vi "detector-init.vi"(5 "Cooling Set":T1={"iDus"=TRUE, "idus-temp"=-90, "Newton"=TRUE, "newton-temp"=-70, "Clara"=TRUE, "clara-temp"=-55, "Xeva"=TRUE, "xeva-temp"=-55} {"xeva-temp" min=-55 max=20 step=5; "clara-temp" min=-55 max=20 step=5; "newton-temp" min=-90 max=20 step=5; "idus-temp" min=-90 max=20 step=5}) -> (0 "Status":T3={"Newton Init"=FALSE, "Newton Cooling"=FALSE, "Newton Parameters "=FALSE, "iDus Init"=FALSE, "iDus Cooling"=FALSE, "iDus Parameters"=FALSE, "Clara Init"=FALSE, "Clara Cooling"=FALSE, "Clara Parameters"=FALSE, "Newton Cooler StatusCode"=enum."DRV_TEMPERATURE_NOT_SUPPORTED", "iDus Cooler StatusCode"=enum."DRV_TEMPERATURE_NOT_SUPPORTED", "Clara Cooler StatusCode"=enum."DRV_TEMPERATURE_NOT_SUPPORTED"} caption="Status Cluster", 1 "cameras initialized":bool, 2 "Handle Cluster":cluster{"iDus":i32, "Newton":i32, "Clara":i32}, 3 "Detector Output Values":cluster{"iDus":i32, "Newton":i32, "Clara":i32}={"iDus"=25, "Newton"=25, "Clara"=25} caption="Detector Temperature Cluster")   [LabVIEW 2015]
uses:
  <userlib>/atmcd32d.llb/Error Code Enum typedef.ctl
  <userlib>/atmcd32d.llb/ReadMode_mode typedef.ctl
  <userlib>/atmcd32d.llb/AcquisitionMode_mode typedef.ctl
  <userlib>/atmcd32d.llb/TriggerMode_mode typedef.ctl
  <userlib>/atmcd32d.llb/HSSpeed_type typedef.ctl
  <userlib>/atmcd32d.llb/OutputAmplifier_type typedef.ctl
panel:
  out "Clara Error":errorcluster
  out "iDus Error":errorcluster
  out "Newton Error":errorcluster
  out "totalCameras":i32
  # "Init"
  # "Cooling"
  # "Parameters"
  # "Newton"
  # "iDus"
  # "Clara"
  # "Clara"
  # "iDus"
  # "Newton"
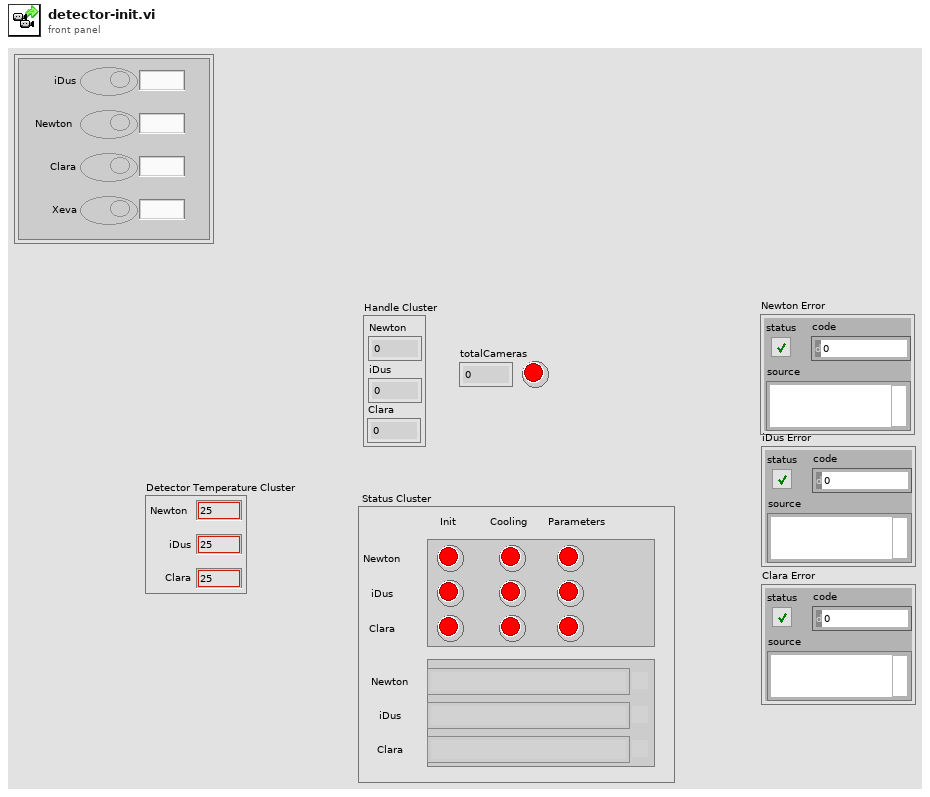
[diagram p1: front panel]
types:
  T1 = cluster{"iDus":bool, "idus-temp":i32, "Newton":bool, "newton-temp":i32, "Clara":bool, "clara-temp":i32, "Xeva":bool, "xeva-temp":i32}
  T2 = typedef "Error Code Enum typedef.ctl" = enum32{"N/A (0)", "DRV_ERROR_CODES", "DRV_SUCCESS", "DRV_VXDNOTINSTALLED", "DRV_ERROR_SCAN", "DRV_ERROR_CHECK_SUM", "DRV_ERROR_FILELOAD", "DRV_UNKNOWN_FUNC", "DRV_ERROR_VXD_INIT", "DRV_ERROR_ADDRESS", "DRV_ERROR_PAGELOCK", "DRV_ERROR_PAGEUNLOCK", "DRV_ERROR_BOARDTEST", "DRV_ERROR_ACK", "DRV_ERROR_UP_FIFO", "DRV_ERROR_PATTERN", "N/A (16)", "DRV_ACQUISITION_ERRORS", "DRV_ACQ_BUFFER", "DRV_ACQ_DOWNFIFO_FULL", "DRV_PROC_UNKONWN_INSTRUCTION", "DRV_ILLEGAL_OP_CODE", "DRV_KINETIC_TIME_NOT_MET", "DRV_ACCUM_TIME_NOT_MET", "DRV_NO_NEW_DATA", "N/A (25)", "DRV_SPOOLERROR", "N/A (27)", "N/A (28)", "N/A (29)", "N/A (30)", "N/A (31)", "N/A (32)", "DRV_TEMPERATURE_CODES", "DRV_TEMPERATURE_OFF", "DRV_TEMPERATURE_NOT_STABILIZED", "DRV_TEMPERATURE_STABILIZED", "DRV_TEMPERATURE_NOT_REACHED", "DRV_TEMPERATURE_OUT_RANGE", "DRV_TEMPERATURE_NOT_SUPPORTED", "DRV_TEMPERATURE_DRIFT", "N/A (41)", "N/A (42)", "N/A (43)", "N/A (44)", "N/A (45)", "N/A (46)", "N/A (47)", "N/A (48)", "DRV_GENERAL_ERRORS", "DRV_INVALID_AUX", "DRV_COF_NOTLOADED", "DRV_FPGAPROG", "DRV_FLEXERROR", "DRV_GPIBERROR", "N/A (55)", "N/A (56)", "N/A (57)", "N/A (58)", "N/A (59)", "N/A (60)", "N/A (61)", "N/A (62)", "N/A (63)", "DRV_DATATYPE", "DRV_DRIVER_ERRORS", "DRV_P1INVALID", "DRV_P2INVALID", "DRV_P3INVALID", "DRV_P4INVALID", "DRV_INIERROR", "DRV_COFERROR", "DRV_ACQUIRING", "DRV_IDLE", "DRV_TEMPCYCLE", "DRV_NOT_INITIALIZED", "DRV_P5INVALID", "DRV_P6INVALID", "DRV_INVALID_MODE", "DRV_INVALID_FILTER", "DRV_I2CERRORS", "DRV_I2CDEVNOTFOUND", "DRV_I2CTIMEOUT", "DRV_P7INVALID", "N/A (84)", "N/A (85)", "N/A (86)", "N/A (87)", "N/A (88)", "N/A (89)", "DRV_IOCERROR", "DRV_VRMVERSIONERROR"}
  T3 = cluster{"Newton Init":bool, "Newton Cooling":bool, "Newton Parameters ":bool, "iDus Init":bool, "iDus Cooling":bool, "iDus Parameters":bool, "Clara Init":bool, "Clara Cooling":bool, "Clara Parameters":bool, "Newton Cooler StatusCode":T2, "iDus Cooler StatusCode":T2, "Clara Cooler StatusCode":T2}
  T4 = cluster{"iDus Init":bool, "Newton Init":bool, "iDus Cooling":bool, "Newton Cooling":bool, "Clara Init":bool, "Clara Cooling":bool, "iDus Parameters":bool, "Newton Parameters ":bool, "Clara Parameters":bool, "Newton Cooler StatusCode":T2, "iDus Cooler StatusCode":T2, "Clara Cooler StatusCode":T2}
  T5 = cluster{"InGaAs Handle":i32, "CCD Handle":i32, "Clara Handle":i32}
  T6 = typedef "TriggerMode_mode typedef.ctl" = enum16{"Internal", "External", "N/A (2)", "N/A (3)", "N/A (4)", "N/A (5)", "External Start", "External Exposure (Bulb)", "N/A (8)", "External FVB EM", "Software", "N/A (11)", "External Charge Shifting"}
  T7 = typedef "AcquisitionMode_mode typedef.ctl" = enum16{"Reserved (0)", "Single Scan", "Accumulate", "Kinetics", "Fast Kinetics", "Run Till Abort", "Reserved (6)", "Reserved (7)", "Reserved (8)", "Time Delayed Integration"}
  T8 = typedef "ReadMode_mode typedef.ctl" = enum16{"Full Vertical Binning", "Multi-Track", "Random-Track", "Single-Track", "Image"}
  T9 = typedef "HSSpeed_type typedef.ctl" = enum16{"EM Amp", "Conventional Amp"}
  T10 = typedef "OutputAmplifier_type typedef.ctl" = enum16{"Standard EMCCD gain register", "Conventional CCD register"}
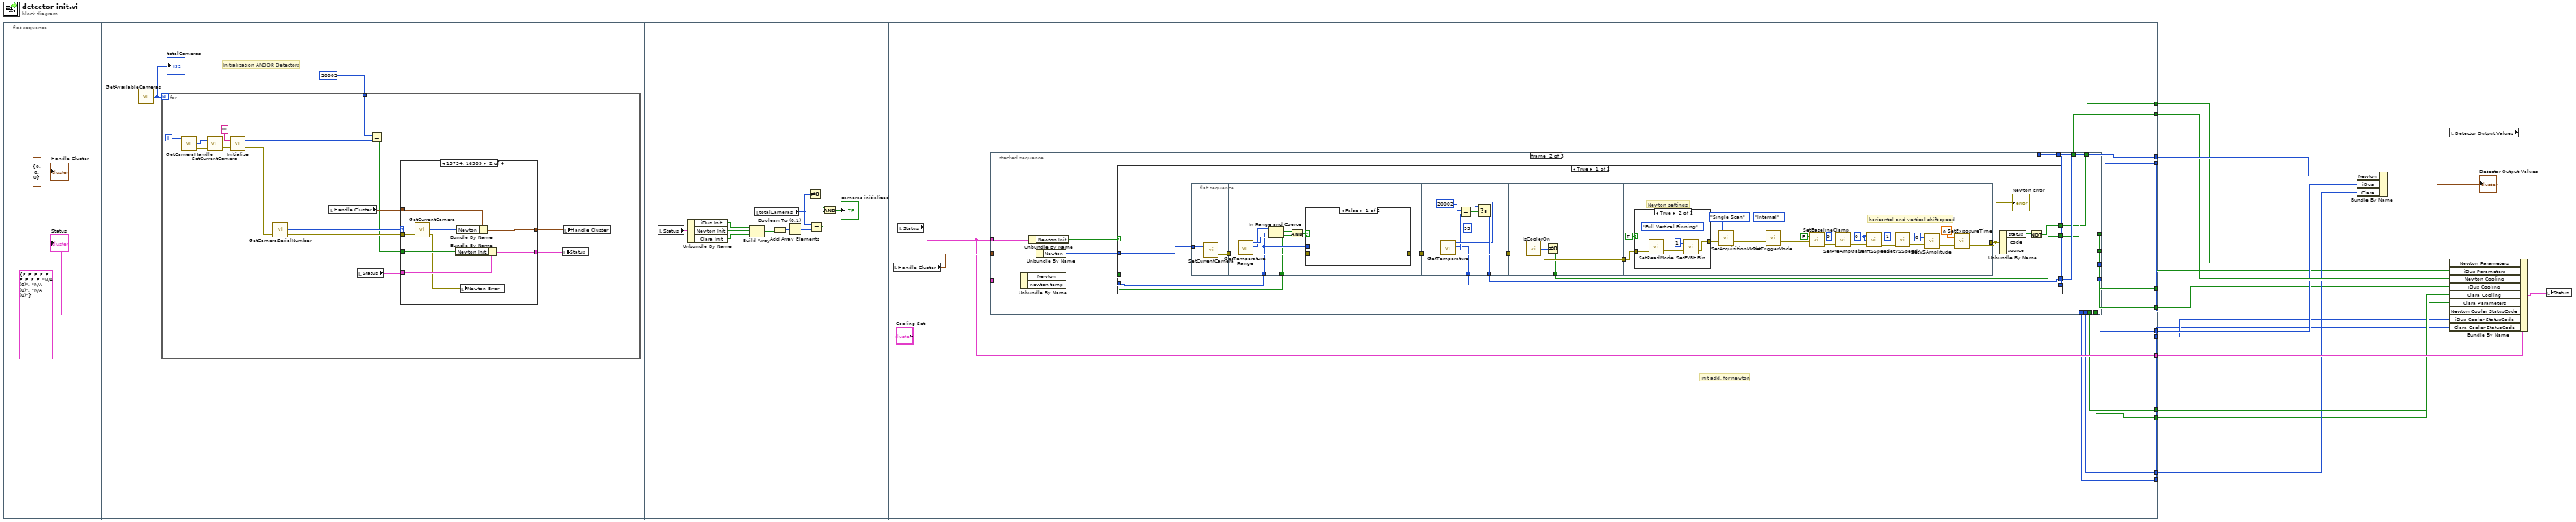
[diagram p0: block diagram]
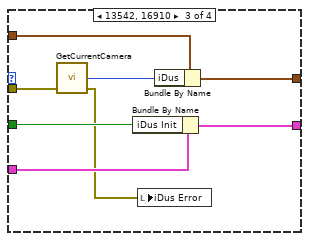
[diagram p3: hidden frame]
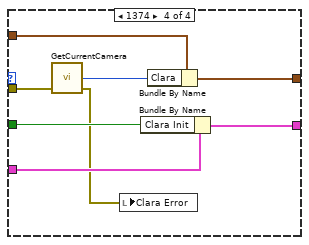
[diagram p4: hidden frame]
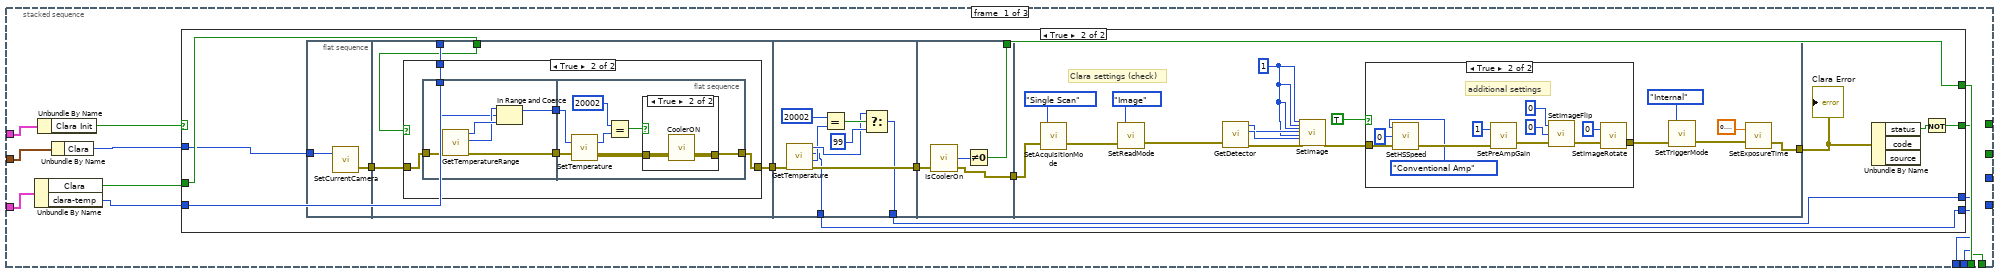
[diagram p5: hidden frame]
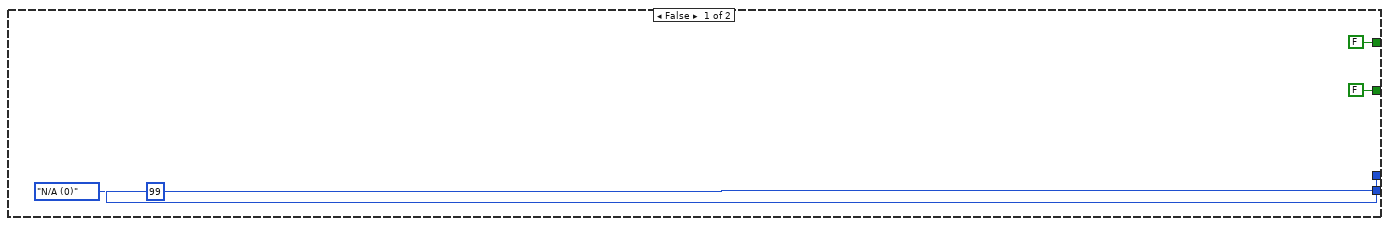
[diagram p6: hidden frame]
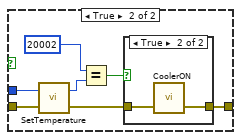
[diagram p10: hidden frame]
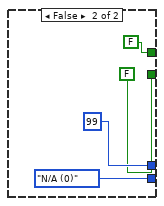
[diagram p13: hidden frame]
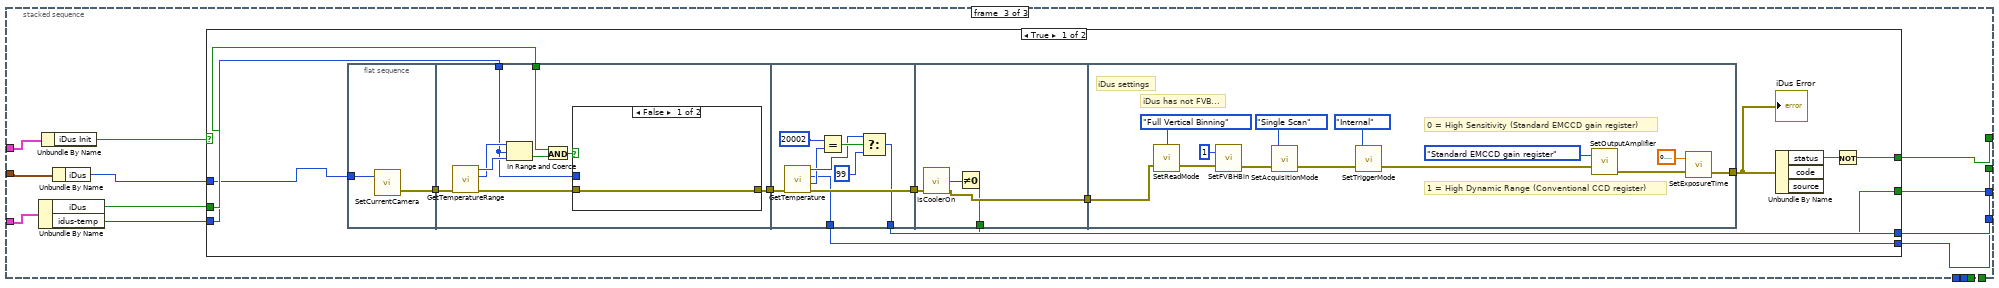
[diagram p14: hidden frame]
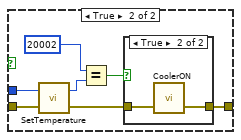
[diagram p15: hidden frame]
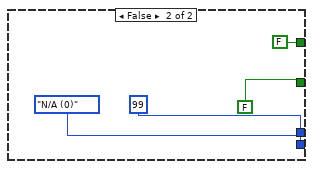
[diagram p17: hidden frame]
diagram:
  n1 = flat-sequence {
    tunnel: [w87] -> w13
    tunnel: [w85] -> w15
    tunnel: [w84] -> w12
    tunnel: [w77] -> w14
    tunnel: [w79] -> w9
    tunnel: [w75] -> w8
    tunnel: [w83] -> w7
    tunnel: [w78] -> w6
    tunnel: [w74] -> w5
    tunnel: [w82] -> w4
    tunnel: [w81] -> w3
    tunnel: [w80] -> w2
    tunnel: [w76] -> w1
    frame #0 {
      "Status" <- T4 {"iDus Init"=FALSE, "Newton Init"=FALSE, "iDus Cooling"=FALSE, "Newton Cooling"=FALSE, "Clara Init"=FALSE, "Clara Cooling"=FALSE, "iDus Parameters"=FALSE, "Newton Parameters "=FALSE, "Clara Parameters"=FALSE, "Newton Cooler StatusCode"=enum."N/A (0)", "iDus Cooler StatusCode"=enum."N/A (0)", "Clara Cooler StatusCode"=enum."N/A (0)"} ("Status")
      "Handle Cluster" <- T5 {"InGaAs Handle"=0, "CCD Handle"=0, "Clara Handle"=0} ("Handle Cluster")
    }
    frame #1 {
      # "Initialization ANDOR Detectors"
      n2 = call <userlib>:"GetAvailableCameras.vi"() -> ("totalCameras"=w20:i32)  [unwired: 3 in, 2 out]
      "totalCameras" <- w20
      n3 = for {
        N: w20 -> [_]
        tunnel: 20002 -> [w33]
        i -> [w28]
        n4 = call <userlib>:"GetCameraHandle.vi"("cameraIndex"=w28) -> ("error out"=w31:errorcluster, "cameraHandle"=w32:i32)  [unwired: 2 in, 1 out]
        n5 = call <userlib>:"SetCurrentCamera.vi"("error in (no error)"=w31, "cameraHandle"=w32) -> ("error out"=w30:errorcluster)  [unwired: 1 out]
        n6 = call <userlib>:"Initialize.vi"("error in (no error)"=w30, "directory (\"\")"="" ("directory (\"\")")) -> ("error out"=w29:errorcluster, "DLL error code"=w34:u32)
        n7 = call <userlib>:"GetCameraSerialNumber.vi"("error in (no error)"=w29) -> ("error out"=w25:errorcluster, "number"=w27:i32)  [unwired: 2 in, 1 out]
        n8 = local read "Handle Cluster"() -> (w26:cluster{"iDus":i32, "Newton":i32, "Clara":i32})
        n9 = local read "Status"() -> (w23:T3)
        n10 = Equal?(x=w33, y=w34) -> (x = y?=w21:bool)
        n11 = case shown="13734, 16909" w27 {
          tunnel: w26 -> [w37 w45 w50 w61]
          tunnel: w25 -> [_ w43 w53 w55]
          tunnel: [w37 w42 w51 w60] -> w24
          tunnel: w23 -> [w36 w41 w49 w58]
          tunnel: [w36 w40 w48 w57] -> w22
          tunnel: w21 -> [_ w39 w47 w56]
          frame 0, Default {
          }
          frame 13734, 16909 {
            n12 = call <userlib>:"GetCurrentCamera.vi"("error in (no error)"=w43) -> ("error out"=w38:errorcluster, "cameraHandle"=w44:i32)  [unwired: 2 in, 1 out]
            n13 = Bundle By Name(cluster=w41, "Newton Init"=w39) -> (w40:T3)
            n14 = Bundle By Name(cluster=w45, "Newton"=w44) -> (w42:cluster{"iDus":i32, "Newton":i32, "Clara":i32})
            n15 = local write "Newton Error"(w38) -> ()
          }
          frame 13542, 16910 {
            n16 = call <userlib>:"GetCurrentCamera.vi"("error in (no error)"=w53) -> ("error out"=w46:errorcluster, "cameraHandle"=w52:i32)  [unwired: 2 in, 1 out]
            n17 = Bundle By Name(cluster=w49, "iDus Init"=w47) -> (w48:T3)
            n18 = local write "iDus Error"(w46) -> ()
            n19 = Bundle By Name(cluster=w50, "iDus"=w52) -> (w51:cluster{"iDus":i32, "Newton":i32, "Clara":i32})
          }
          frame 1374 {
            n20 = call <userlib>:"GetCurrentCamera.vi"("error in (no error)"=w55) -> ("error out"=w54:errorcluster, "cameraHandle"=w59:i32)  [unwired: 2 in, 1 out]
            n21 = local write "Clara Error"(w54) -> ()
            n22 = Bundle By Name(cluster=w58, "Clara Init"=w56) -> (w57:T3)
            n23 = Bundle By Name(cluster=w61, "Clara"=w59) -> (w60:cluster{"iDus":i32, "Newton":i32, "Clara":i32})
          }
        }
        n24 = local write "Status"(w22) -> ()
        n25 = local write "Handle Cluster"(w24) -> ()
      }
    }
    frame #2 {
      n26 = local read "Status"() -> (w72:T3)
      n27 = Unbundle By Name(w72) -> ("iDus Init"=w71:bool, "Newton Init"=w70:bool, "Clara Init"=w69:bool)
      n28 = Build Array(w71, w70, w69) -> (w68:bool[])
      n29 = local read "totalCameras"() -> (w65:i32)
      n30 = Boolean To (0,1)(Boolean=w68) -> (0, 1=w67:i16[])
      n31 = Add Array Elements(numeric array=w67) -> (sum=w66:i16)
      n32 = Not Equal To 0?(x=w65) -> (x != 0?=w63:bool)
      n33 = Equal?(x=w65, y=w66) -> (x = y?=w64:bool)
      n34 = And(x=w63, y=w64) -> (x .and. y?=→"cameras initialized":bool)
    }
    frame #3 {
      # "init add. for newton"
      n35 = local read "Handle Cluster"() -> (w86:cluster{"iDus":i32, "Newton":i32, "Clara":i32})
      n36 = local read "Status"() -> (w85:T3)
      n37 = stacked-sequence {
        tunnel: [_ w194 _] -> w87
        tunnel: w86 -> [w89 w191 w273]
        tunnel: w85 -> [w90 w190 w274]
        tunnel: [_ w189 _] -> w84
        tunnel: "Cooling Set" -> [w88 w186 w272]
        tunnel: [_ w185 _] -> w83
        tunnel: [_ w184 _] -> w82
        tunnel: [_ _ w278] -> w81
        tunnel: [_ _ w277] -> w80
        tunnel: [_ _ w276] -> w79
        tunnel: [_ _ w275] -> w78
        tunnel: [w94 _ _] -> w77
        tunnel: [w93 _ _] -> w76
        tunnel: [w92 _ _] -> w75
        tunnel: [w91 _ _] -> w74
        frame #0 {
          n38 = Unbundle By Name(w88) -> ("Clara"=w96:bool, "clara-temp"=w95:i32)
          n39 = Unbundle By Name(w90) -> ("Clara Init"=w98:bool)
          n40 = Unbundle By Name(w89) -> ("Clara"=w97:i32)
          n41 = case shown="True" w98 {
            tunnel: w95 -> [_ w111]
            tunnel: w96 -> [_ w110]
            tunnel: w97 -> [_ w109]
            tunnel: [FALSE w108] -> w94
            tunnel: [u32 99 ("status") w107] -> w92
            tunnel: [Error_Code_Enum_typedef."N/A (0)" ("status") w106] -> w91
            tunnel: [FALSE w103] -> w93
            frame False {
            }
            frame True {
              n42 = flat-sequence {
                tunnel: [w117] -> w115
                tunnel: w109 -> [w116]
                tunnel: [w121] -> w114
                tunnel: w110 -> [w120]
                tunnel: w111 -> [w118]
                tunnel: w115 -> [w119]
                tunnel: w114 -> [w151]
                tunnel: [w150] -> w113
                tunnel: [w147] -> w107
                tunnel: [w143] -> w106
                tunnel: w113 -> [w155]
                tunnel: [w153] -> w112
                tunnel: [w152] -> w108
                tunnel: w112 -> [w164]
                tunnel: [w169] -> w105
                frame #0 {
                  n43 = call <userlib>:"SetCurrentCamera.vi"("cameraHandle"=w116) -> ("error out"=w117:errorcluster)  [unwired: 1 in, 1 out]
                }
                frame #1 {
                  n44 = case shown="True" w120 {
                    tunnel: [w122 w124] -> w121
                    tunnel: w119 -> [w122 w125]
                    tunnel: w118 -> [_ w123]
                    frame False {
                    }
                    frame True {
                      n45 = flat-sequence {
                        tunnel: [w131] -> w127
                        tunnel: [w130] -> w126
                        tunnel: w125 -> [w129]
                        tunnel: w123 -> [w128]
                        tunnel: [w139] -> w124
                        tunnel: w127 -> [w139]
                        tunnel: w126 -> [w134]
                        frame #0 {
                          n46 = call <userlib>:"GetTemperatureRange.vi"("error in (no error)"=w129) -> ("error out"=w131:errorcluster, "maxTemp"=w132:i32, "minTemp"=w133:i32)  [unwired: 3 in, 1 out]
                          n47 = In Range and Coerce(upper limit=w132, x=w128, lower limit=w133) -> (coerced(x)=w130:i32)  [unwired: 1 out]
                        }
                        frame #1 {
                          n48 = call <userlib>:"SetTemperature.vi"("temperature"=w134) -> ("error out"=w137:errorcluster, "DLL error code"=w135:u32)  [unwired: 1 in]
                          n49 = Equal?(x=20002, y=w135) -> (x = y?=w136:bool)
                          n50 = case shown="True" w136 {
                            tunnel: [w140 w142] -> _
                            tunnel: w137 -> [w140 w141]
                            frame False {
                            }
                            frame True {
                              n51 = call <userlib>:"CoolerON.vi"("error in (no error)"=w141) -> ("error out"=w142:errorcluster)  [unwired: 1 in, 1 out]
                            }
                          }
                        }
                      }
                    }
                  }
                }
                frame #2 {
                  n52 = call <userlib>:"GetTemperature.vi"("error in (no error)"=w151) -> ("error out"=w150:errorcluster, "DLL error code"=w144:u32, "status"=w143:T2, "temperature"=w145:i32)  [unwired: 3 in]
                  n53 = Equal?(x=20002, y=w144) -> (x = y?=w148:bool)
                  n54 = Select(t=w145, s=w148, f=99) -> (s? t:f=w147:i32)
                }
                frame #3 {
                  n55 = call <userlib>:"IsCoolerOn.vi"("error in (no error)"=w155) -> ("error out"=w153:errorcluster, "coolerStatus"=w154:i32)  [unwired: 2 in, 1 out]
                  n56 = Not Equal To 0?(x=w154) -> (x != 0?=w152:bool)
                }
                frame #4 {
                  w157 = 1 ("hbin")
                  # "Clara settings (check)"
                  n57 = call <userlib>:"SetAcquisitionMode.vi"("error in (no error)"=w164, "mode"=AcquisitionMode_mode_typedef."Single Scan") -> ("error out"=w163:errorcluster)  [unwired: 1 out]
                  n58 = call <userlib>:"SetReadMode.vi"("error in (no error)"=w163, "mode"=ReadMode_mode_typedef."Image") -> ("error out"=w156:errorcluster)  [unwired: 1 out]
                  n59 = call <userlib>:"GetDetector.vi"("error in (no error)"=w156) -> ("error out"=w162:errorcluster, "ypixels"=w161:i32, "xpixels"=w160:i32)  [unwired: 3 in, 1 out]
                  n60 = call <userlib>:"SetImage.vi"("hbin"=w157, "vbin"=w157, "hstart"=w157, "hend"=w160, "vstart"=w157, "vend"=w161, "error in (no error)"=w162) -> ("error out"=w159:errorcluster)  [unwired: 19 in, 1 out]
                  n61 = case shown="True" TRUE {
                    tunnel: [w172 w177] -> w166
                    tunnel: w159 -> [w172 w175]
                    frame False {
                    }
                    frame True {
                      # "additional settings"
                      n62 = call <userlib>:"SetHSSpeed.vi"("error in (no error)"=w175, "index"=0, "type"=HSSpeed_type_typedef."Conventional Amp") -> ("error out"=w176:errorcluster)  [unwired: 1 in, 1 out]
                      n63 = call <userlib>:"SetPreAmpGain.vi"("error in (no error)"=w176, "index"=1) -> ("error out"=w182:errorcluster)  [unwired: 1 out]
                      n64 = call <userlib>:"SetImageFlip.vi"("error in (no error)"=w182, "VFlip"=0, "HFlip"=0) -> ("error out"=w179:errorcluster)  [unwired: 1 in, 1 out]
                      n65 = call <userlib>:"SetImageRotate.vi"("error in (no error)"=w179, "Rotate"=0) -> ("error out"=w177:errorcluster)  [unwired: 1 out]
                    }
                  }
                  n66 = call <userlib>:"SetTriggerMode.vi"("error in (no error)"=w166, "mode"=TriggerMode_mode_typedef."Internal") -> ("error out"=w165:errorcluster)  [unwired: 1 out]
                  n67 = call <userlib>:"SetExposureTime.vi"("error in (no error)"=w165, "time"=sgl 0.2) -> ("error out"=w169:errorcluster)  [unwired: 1 out]
                }
              }
              n68 = Unbundle By Name(w105) -> ("status"=w104:bool)  [unwired: 2 out]
              n69 = Not(x=w104) -> (.not. x?=w103:bool)
              "Clara Error" <- w105
            }
          }
        }
        frame #1 {
          n70 = Unbundle By Name(w186) -> ("Newton"=w188:bool, "newton-temp"=w187:i32)
          n71 = Unbundle By Name(w190) -> ("Newton Init"=w193:bool)
          n72 = Unbundle By Name(w191) -> ("Newton"=w192:i32)
          n73 = case shown="True" w193 {
            tunnel: w188 -> [w204 _]
            tunnel: w187 -> [w203 _]
            tunnel: [w195 99 ("f")] -> w194
            tunnel: w192 -> [w201 _]
            tunnel: [w200 FALSE] -> w189
            tunnel: [w199 Error_Code_Enum_typedef."N/A (0)" ("status")] -> w185
            tunnel: [w197 FALSE] -> w184
            frame True {
              n74 = flat-sequence {
                tunnel: [w209] -> w207
                tunnel: w201 -> [w208]
                tunnel: [w214] -> w206
                tunnel: w204 -> [w211]
                tunnel: w203 -> [w213]
                tunnel: w207 -> [w210]
                tunnel: w206 -> [w238]
                tunnel: [w237] -> w205
                tunnel: [w234] -> w195
                tunnel: [w230] -> w199
                tunnel: w205 -> [w242]
                tunnel: [w241] -> w202
                tunnel: [w239] -> w200
                tunnel: w202 -> [w245]
                tunnel: [w248] -> w196
                frame #0 {
                  n75 = call <userlib>:"SetCurrentCamera.vi"("cameraHandle"=w208) -> ("error out"=w209:errorcluster)  [unwired: 1 in, 1 out]
                }
                frame #1 {
                  n76 = call <userlib>:"GetTemperatureRange.vi"("error in (no error)"=w210) -> ("error out"=w215:errorcluster, "maxTemp"=w216:i32, "minTemp"=w217:i32)  [unwired: 3 in, 1 out]
                  n77 = In Range and Coerce(upper limit=w216, x=w213, lower limit=w217) -> (In Range?=w212:bool)  [unwired: 1 out]
                  n78 = And(x=w211, y=w212) -> (x .and. y?=w218:bool)
                  n79 = case shown="False" w218 {
                    tunnel: w213 -> [_ w226]
                    tunnel: w215 -> [w219 w222]
                    tunnel: [w219 w220] -> w214
                    frame False {
                    }
                    frame True {
                      n80 = call <userlib>:"SetTemperature.vi"("error in (no error)"=w222, "temperature"=w226) -> ("error out"=w223:errorcluster, "DLL error code"=w225:u32)
                      n81 = Equal?(x=20002, y=w225) -> (x = y?=w224:bool)
                      n82 = case shown="True" w224 {
                        tunnel: [w227 w229] -> w220
                        tunnel: w223 -> [w227 w228]
                        frame False {
                        }
                        frame True {
                          n83 = call <userlib>:"CoolerON.vi"("error in (no error)"=w228) -> ("error out"=w229:errorcluster)  [unwired: 1 in, 1 out]
                        }
                      }
                    }
                  }
                }
                frame #2 {
                  n84 = call <userlib>:"GetTemperature.vi"("error in (no error)"=w238) -> ("error out"=w237:errorcluster, "DLL error code"=w231:u32, "status"=w230:T2, "temperature"=w232:i32)  [unwired: 3 in]
                  n85 = Equal?(x=20002, y=w231) -> (x = y?=w235:bool)
                  n86 = Select(t=w232, s=w235, f=99) -> (s? t:f=w234:i32)
                }
                frame #3 {
                  n87 = call <userlib>:"IsCoolerOn.vi"("error in (no error)"=w242) -> ("error out"=w241:errorcluster, "coolerStatus"=w240:i32)  [unwired: 2 in, 1 out]
                  n88 = Not Equal To 0?(x=w240) -> (x != 0?=w239:bool)
                }
                frame #4 {
                  w256 = 0 ("index")
                  # "horizontal and vertical shift speed"
                  # "Newton settings"
                  n89 = case shown="True" TRUE {
                    tunnel: w245 -> [w262 w264]
                    tunnel: [w262 w263] -> w244
                    frame False {
                    }
                    frame True {
                      n90 = call <userlib>:"SetReadMode.vi"("error in (no error)"=w264, "mode"=ReadMode_mode_typedef."Full Vertical Binning") -> ("error out"=w266:errorcluster)  [unwired: 1 out]
                      n91 = call <userlib>:"SetFVBHBin.vi"("error in (no error)"=w266, "bin"=1) -> ("error out"=w263:errorcluster)  [unwired: 1 out]
                    }
                  }
                  n92 = call <userlib>:"SetAcquisitionMode.vi"("error in (no error)"=w244, "mode"=AcquisitionMode_mode_typedef."Single Scan") -> ("error out"=w251:errorcluster)  [unwired: 1 out]
                  n93 = call <userlib>:"SetTriggerMode.vi"("error in (no error)"=w251, "mode"=TriggerMode_mode_typedef."Internal") -> ("error out"=w252:errorcluster)  [unwired: 1 out]
                  n94 = call <userlib>:"SetBaselineClamp.vi"("error in (no error)"=w252, "state"=FALSE) -> ("error out"=w255:errorcluster)  [unwired: 1 out]
                  n95 = call <userlib>:"SetPreAmpGain.vi"("error in (no error)"=w255, "index"=0) -> ("error out"=w258:errorcluster)  [unwired: 1 out]
                  n96 = call <userlib>:"SetHSSpeed.vi"("error in (no error)"=w258, "index"=w256, "type"=w256) -> ("error out"=w259:errorcluster)  [unwired: 1 in, 1 out]
                  n97 = call <userlib>:"SetVSSpeed.vi"("error in (no error)"=w259, "index"=1) -> ("error out"=w261:errorcluster)  [unwired: 1 out]
                  n98 = call <userlib>:"SetVSAmplitude.vi"("error in (no error)"=w261, "amplitude"=0) -> ("error out"=w246:errorcluster)  [unwired: 1 out]
                  n99 = call <userlib>:"SetExposureTime.vi"("error in (no error)"=w246, "time"=sgl 0.2) -> ("error out"=w248:errorcluster)  [unwired: 1 out]
                }
              }
              n100 = Unbundle By Name(w196) -> ("status"=w198:bool)  [unwired: 2 out]
              n101 = Not(x=w198) -> (.not. x?=w197:bool)
              "Newton Error" <- w196
            }
            frame False {
            }
          }
        }
        frame #2 {
          n102 = Unbundle By Name(w272) -> ("iDus"=w280:bool, "idus-temp"=w279:i32)
          n103 = Unbundle By Name(w274) -> ("iDus Init"=w282:bool)
          n104 = Unbundle By Name(w273) -> ("iDus"=w281:i32)
          n105 = case shown="True" w282 {
            tunnel: w280 -> [w292 _]
            tunnel: w279 -> [w291 _]
            tunnel: [w290 99 ("f")] -> w276
            tunnel: w281 -> [w288 _]
            tunnel: [w287 FALSE] -> w277
            tunnel: [w286 Error_Code_Enum_typedef."N/A (0)" ("status")] -> w275
            tunnel: [w283 FALSE] -> w278
            frame True {
              n106 = flat-sequence {
                tunnel: [w297] -> w295
                tunnel: w288 -> [w296]
                tunnel: [w302] -> w294
                tunnel: w292 -> [w299]
                tunnel: w291 -> [w301]
                tunnel: w295 -> [w298]
                tunnel: w294 -> [w326]
                tunnel: [w325] -> w293
                tunnel: [w322] -> w290
                tunnel: [w318] -> w286
                tunnel: w293 -> [w330]
                tunnel: [w328] -> w289
                tunnel: [w327] -> w287
                tunnel: [w332] -> w284
                tunnel: w289 -> [w331]
                frame #0 {
                  n107 = call <userlib>:"SetCurrentCamera.vi"("cameraHandle"=w296) -> ("error out"=w297:errorcluster)  [unwired: 1 in, 1 out]
                }
                frame #1 {
                  n108 = call <userlib>:"GetTemperatureRange.vi"("error in (no error)"=w298) -> ("error out"=w303:errorcluster, "maxTemp"=w304:i32, "minTemp"=w305:i32)  [unwired: 3 in, 1 out]
                  n109 = In Range and Coerce(upper limit=w304, x=w301, lower limit=w305) -> (In Range?=w300:bool)  [unwired: 1 out]
                  n110 = And(x=w299, y=w300) -> (x .and. y?=w306:bool)
                  n111 = case shown="False" w306 {
                    tunnel: w301 -> [_ w314]
                    tunnel: w303 -> [w307 w310]
                    tunnel: [w307 w308] -> w302
                    frame False {
                    }
                    frame True {
                      n112 = call <userlib>:"SetTemperature.vi"("error in (no error)"=w310, "temperature"=w314) -> ("error out"=w311:errorcluster, "DLL error code"=w313:u32)
                      n113 = Equal?(x=20002, y=w313) -> (x = y?=w312:bool)
                      n114 = case shown="True" w312 {
                        tunnel: [w315 w317] -> w308
                        tunnel: w311 -> [w315 w316]
                        frame False {
                        }
                        frame True {
                          n115 = call <userlib>:"CoolerON.vi"("error in (no error)"=w316) -> ("error out"=w317:errorcluster)  [unwired: 1 in, 1 out]
                        }
                      }
                    }
                  }
                }
                frame #2 {
                  n116 = call <userlib>:"GetTemperature.vi"("error in (no error)"=w326) -> ("error out"=w325:errorcluster, "DLL error code"=w319:u32, "status"=w318:T2, "temperature"=w320:i32)  [unwired: 3 in]
                  n117 = Equal?(x=20002, y=w319) -> (x = y?=w323:bool)
                  n118 = Select(t=w320, s=w323, f=99) -> (s? t:f=w322:i32)
                }
                frame #3 {
                  n119 = call <userlib>:"IsCoolerOn.vi"("error in (no error)"=w330) -> ("error out"=w328:errorcluster, "coolerStatus"=w329:i32)  [unwired: 2 in, 1 out]
                  n120 = Not Equal To 0?(x=w329) -> (x != 0?=w327:bool)
                }
                frame #4 {
                  # "iDus has not FVB..."
                  # "iDus settings"
                  # "1 = High Dynamic Range (Conventional CCD register)"
                  # "0 = High Sensitivity (Standard EMCCD gain register)"
                  n121 = call <userlib>:"SetReadMode.vi"("error in (no error)"=w331, "mode"=ReadMode_mode_typedef."Full Vertical Binning") -> ("error out"=w337:errorcluster)  [unwired: 1 out]
                  n122 = call <userlib>:"SetFVBHBin.vi"("error in (no error)"=w337, "bin"=1) -> ("error out"=w339:errorcluster)  [unwired: 1 out]
                  n123 = call <userlib>:"SetAcquisitionMode.vi"("error in (no error)"=w339, "mode"=AcquisitionMode_mode_typedef."Single Scan") -> ("error out"=w336:errorcluster)  [unwired: 1 out]
                  n124 = call <userlib>:"SetTriggerMode.vi"("error in (no error)"=w336, "mode"=TriggerMode_mode_typedef."Internal") -> ("error out"=w340:errorcluster)  [unwired: 1 out]
                  n125 = call <userlib>:"SetOutputAmplifier.vi"("error in (no error)"=w340, "type"=OutputAmplifier_type_typedef."Standard EMCCD gain register") -> ("error out"=w342:errorcluster)  [unwired: 1 out]
                  n126 = call <userlib>:"SetExposureTime.vi"("error in (no error)"=w342, "time"=sgl 0.2) -> ("error out"=w332:errorcluster)  [unwired: 1 out]
                }
              }
              n127 = Unbundle By Name(w284) -> ("status"=w285:bool)  [unwired: 2 out]
              n128 = Not(x=w285) -> (.not. x?=w283:bool)
              "iDus Error" <- w284
            }
            frame False {
            }
          }
        }
      }
    }
  }
  n129 = Bundle By Name(cluster=w15, "Newton Parameters"=w4, "iDus Parameters"=w3, "Newton Cooling"=w12, "iDus Cooling"=w2, "Clara Cooling"=w14, "Clara Parameters"=w1, "Newton Cooler StatusCode"=w7, "iDus Cooler StatusCode"=w6, "Clara Cooler StatusCode"=w5) -> (w16:T3)
  n130 = local read "Detector Output Values"() -> (w10:cluster{"iDus":i32, "Newton":i32, "Clara":i32})
  n131 = Bundle By Name(cluster=w10, "Newton"=w13, "iDus"=w9, "Clara"=w8) -> (→"Detector Output Values":cluster{"iDus":i32, "Newton":i32, "Clara":i32})
  n132 = local write "Status"(w16) -> ()
